vi "load_name.vi"(8 "error in":errorcluster) -> (0 "error out":errorcluster, 2 "Saving Path Out":path, 3 "Name Out":string)   [LabVIEW 2023]
uses:
  control/global name path.vi
panel:
  in  "Saving Path":path
  in  "Name":string
  in  "Stop":bool
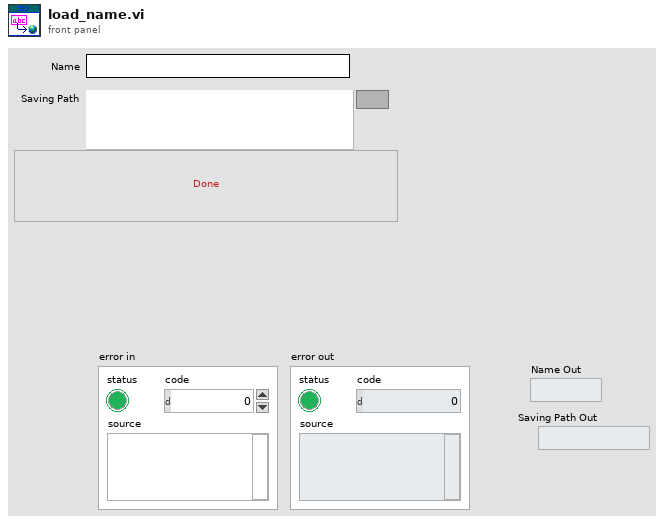
[diagram p1: front panel]
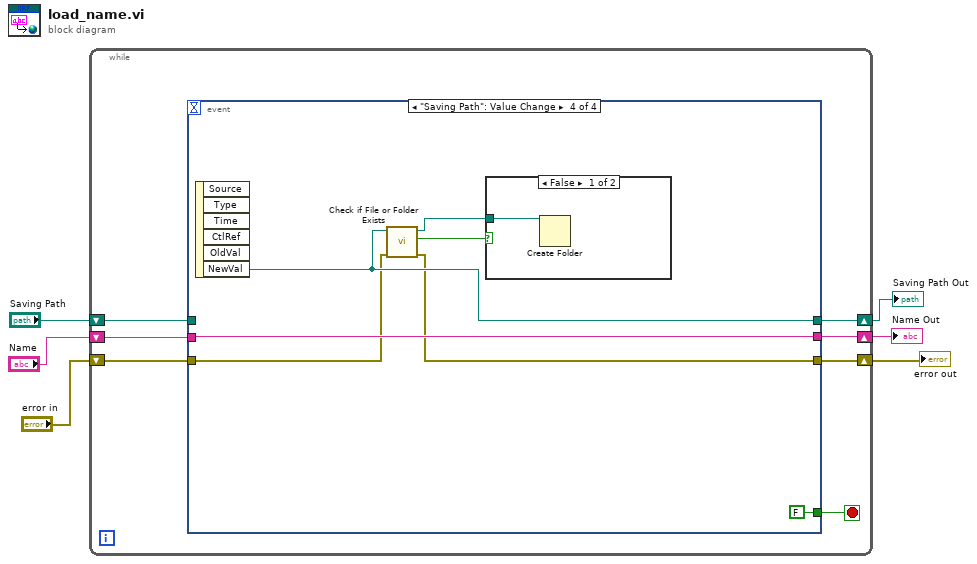
[diagram p0: block diagram]
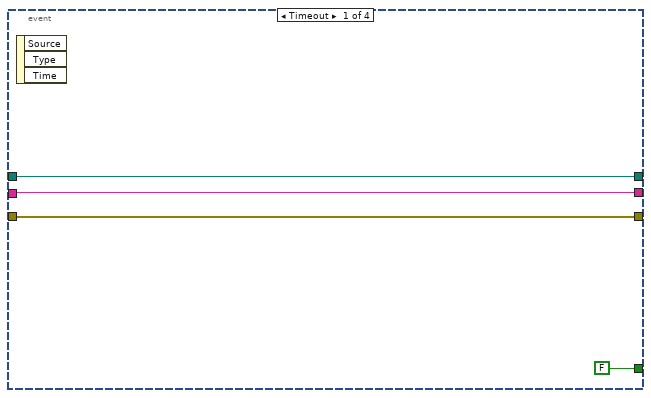
[diagram p2: hidden frame]
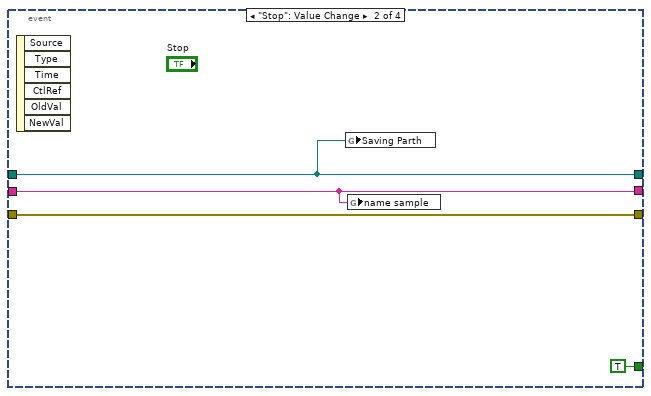
[diagram p3: hidden frame]
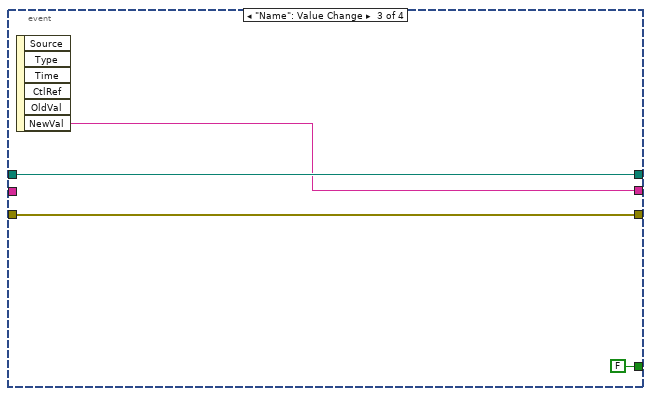
[diagram p4: hidden frame]
diagram:
  n1 = while {
    shift-right: [w11] -> w5
    shift-left: "error in" -> [w12]
    shift-right: [w10] -> w2
    shift-left: "Name" -> [w9]
    shift-right: [w8] -> w1
    shift-left: "Saving Path" -> [w7]
    stop <- w13 stop-if-true
    n2 = event shown="[3] \"Saving Path\": Value Change" {
      selector: _ -> [_ _ _ _]
      dyn-events: _ -> [_ _ _ _]
      timeout: _ -> [_ _ _ _]
      tunnel: [FALSE TRUE FALSE FALSE] -> w13
      tunnel: w12 -> [w16 w21 w24 w29]
      tunnel: [w16 w21 w24 w28] -> w11
      tunnel: [w14 w18 w22 w31] -> w10
      tunnel: w9 -> [w14 w18 _ w31]
      tunnel: [w15 w19 w23 w30] -> w8
      tunnel: w7 -> [w15 w19 w23 _]
      event Timeout {
        n3 = event-data() -> ()  [unwired: 1 in, 3 out]
      }
      event "Stop": Value Change {
        n4 = event-data() -> ()  [unwired: 1 in, 6 out]
        n5 = global write "global name path.vi" "Saving Parth"(w19) -> ()
        n6 = global write "global name path.vi" "name sample"(w18) -> ()
      }
      event "Name": Value Change {
        n7 = event-data() -> ("NewVal"=w22:string)  [unwired: 1 in, 5 out]
      }
      event "Saving Path": Value Change {
        n8 = event-data() -> ("NewVal"=w30:path)  [unwired: 1 in, 5 out]
        n9 = call <vilib>:"Check if File or Folder Exists.vi"("error in (no error)"=w29, "path"=w30) -> ("error out"=w28:errorcluster, "file or folder exists?"=w27:bool, "dup path"=w26:path)  [unwired: 7 in]
        n10 = case shown="False" w27 {
          tunnel: w26 -> [w33 _]
          frame False {
            n11 = Create Folder(path (use dialog)=w33) -> ()  [unwired: 2 in, 3 out]
          }
          frame True {
          }
        }
      }
    }
  }
  "error out" <- w5
  "Name Out" <- w2
  "Saving Path Out" <- w1
